vi "get target by ID.vi"(8 "error in":errorcluster, 10 "UID":string, 11 "full system":T1) -> (0 "error out":errorcluster, 3 "target hierarchy":T1)   [LabVIEW 2013, in "PL_Serialization Interface.lvlib"]
doc: "Searches a flattened instance data hierarhy for a specific target by the UID and returns target data, assuming that the current root element is the system level. If the target is not found, error 538508 is returned."
uses:
  PL_Serialization Interface.lvlib
  <vilib>/NI/Configuration Framework/tree serializer/flat hierarchy.ctl
  <vilib>/NI/Configuration Framework/tree serializer/full hierarchy.ctl
  <vilib>/NI/Configuration Framework/tree serializer/hierarchy element.ctl
  <vilib>/NI/Configuration Framework/tree serializer/instance data.ctl
  <vilib>/NI/Configuration Framework/tree serializer/NISE_CEF_TreeSerializer.lvlib
  <vilib>/NI/Configuration Framework/NISE_CEF_TreeControl.lvlib
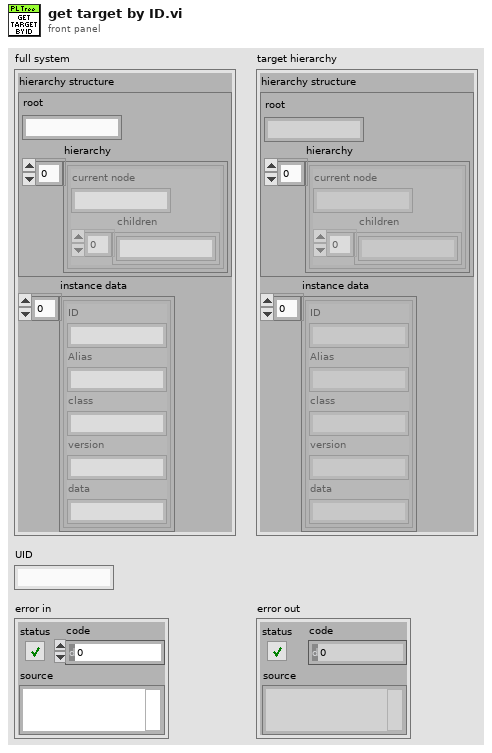
[diagram p1: front panel]
types:
  T1 = typedef "NISE_CEF_TreeSerializer.lvlib/flat hierarchy.ctl" = cluster{"hierarchy structure":T2, "instance data":T4[]}
  T2 = typedef "NISE_CEF_TreeSerializer.lvlib/full hierarchy.ctl" = cluster{"root":string, "hierarchy":T3[]}
  T3 = typedef "NISE_CEF_TreeSerializer.lvlib/hierarchy element.ctl" = cluster{"current node":string, "children":string[]}
  T4 = typedef "NISE_CEF_TreeSerializer.lvlib/instance data.ctl" = cluster{"ID":string, "Alias":string, "class":string, "version":string, "data":string}
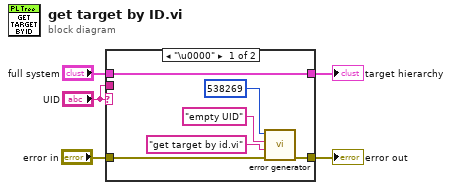
[diagram p0: block diagram]
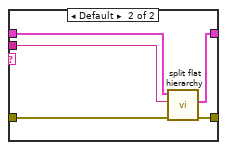
[diagram p2: hidden frame]
diagram:
  n1 = case shown="\"\"" "UID" {
    tunnel: "full system" -> [w11 w16]
    tunnel: "error in" -> [w10 w15]
    tunnel: "UID" -> [_ w14]
    tunnel: [w9 w13] -> w3
    tunnel: [w11 w12] -> w2
    frame "\u0000" {
      n2 = call <vilib>:"error generator.vi"("error in"=w10, "source"="get target by id.vi", "append error message"="empty UID", "error code (0)"=538269) -> ("error out"=w9:errorcluster)  [unwired: 5 in]
    }
    frame Default {
      n3 = call <vilib>:"split flat hierarchy.vi"("error in"=w15, "UID"=w14, "flat hierarchy"=w16) -> ("error out"=w13:errorcluster, "flat hierarchy with UID"=w12:T1)  [unwired: 6 in, 1 out]
    }
  }
  "error out" <- w3
  "target hierarchy" <- w2
